vi "LVDemo2.vi"() -> ()   [LabVIEW 2010]
uses:
  toupcam.dll
  toupcam_labview.dll
panel:
  in  "Tab 2":T1(tab)
  in  "Color Default 2":bool
  in  "Brightness 2":i32(slide) scale=-64.0..64.0
  in  "Contrast 2":i32(slide) scale=-100.0..100.0
  in  "Gamma 2":i32(slide) scale=20.0..180.0
  in  "Hue 2":i32(slide) scale=-180.0..180.0
  in  "Saturation 2":i32(slide) scale=0.0..255.0
  in  "AutoExpo 2":bool
  in  "ExpoDefault 2":bool
  in  "Expotime 2":u32(slide)
  in  "ExpoGain 2":u16(slide)
  in  "AutoWB 2":bool
  in  "WBDefault 2":bool
  in  "Tint 2":i32(slide) scale=200.0..2500.0
  in  "Temp 2":i32(slide) scale=2000.0..15000.0
  in  "Bin/Skip Mode 2":bool
  in  "Chrome/Mono 2":bool
  in  "HFlip 2":bool
  in  "VFlip 2":bool
  in  "Frame Speed 2":u8(slide) scale=0.0..87.0
  in  "Cap Still Image 2":bool
  in  "Still Image Resolution 2":u16(ring)
  in  "Cap Live Image 2":bool
  in  "Live Resolution 2":u16(ring)
  out "Video 2":T2(plugin-control)
  in  "Tab":T1(tab)
  in  "Color Default":bool
  in  "Brightness":i32(slide) scale=-64.0..64.0
  in  "Contrast":i32(slide) scale=-100.0..100.0
  in  "Gamma":i32(slide) scale=20.0..180.0
  in  "Hue":i32(slide) scale=-180.0..180.0
  in  "Saturation":i32(slide) scale=0.0..255.0
  in  "AutoExpo":bool
  in  "ExpoDefault":bool
  in  "Expotime":u32(slide) scale=294.0..2000000.0
  in  "ExpoGain":u16(slide) scale=100.0..300.0
  in  "AutoWB":bool
  in  "WBDefault":bool
  in  "Tint":i32(slide) scale=200.0..2500.0
  in  "Temp":i32(slide) scale=2000.0..15000.0
  in  "Bin/Skip Mode":bool
  in  "Chrome/Mono":bool
  in  "HFlip":bool
  in  "VFlip":bool
  in  "Frame Speed":u8(slide) scale=0.0..6.0
  out "Video":T2(plugin-control)
  in  "Cap Still Image":bool
  in  "Still Image Resolution":u16(ring) items=["2592*1944", "1280*960", "640*480"]
  in  "Cap Live Image":bool
  in  "Stop":bool
  in  "Live Resolution":u16(ring) items=["2592*1944", "1280*960", "640*480"]
  in  "?":enum32{"选项卡 1"}(tab)
  in  "Expotime_def 2":u32
  in  "ExpoGain_def 2":u16
  in  "ExpoGain_Max 2":u16
  in  "ExpoGain_Min 2":u16
  in  "Height 2":i32
  in  "Width 2":i32
  in  "Expotime_Max 2":u32
  in  "Expotime_Min 2":u32
  in  "speed 2":u8
  in  "height22":i32
  in  "width22":i32
  in  "Mode 2":bool
  in  "Expotime_def":u32
  in  "ExpoGain_def":u16
  in  "ExpoGain_Max":u16
  in  "ExpoGain_Min":u16
  in  "Height":i32
  in  "Width":i32
  in  "Expotime_Max":u32
  in  "Expotime_Min":u32
  in  "speed":u8
  in  "height12":i32
  in  "width12":i32
  in  "Mode":bool
  in  "Still_Height 3":i32
  in  "Still_Width 3":i32
  in  "ExpoGain 5":u16
  in  "Expotime 5":u32
  in  "Tint 5":i32
  in  "Temp 5":i32
  in  "ExpoGain 6":u16
  in  "Expotime 6":u32
  in  "Temp 6":i32
  in  "Tint 6":i32
  in  "Still_Width 4":i32
  in  "Still_Height 4":i32
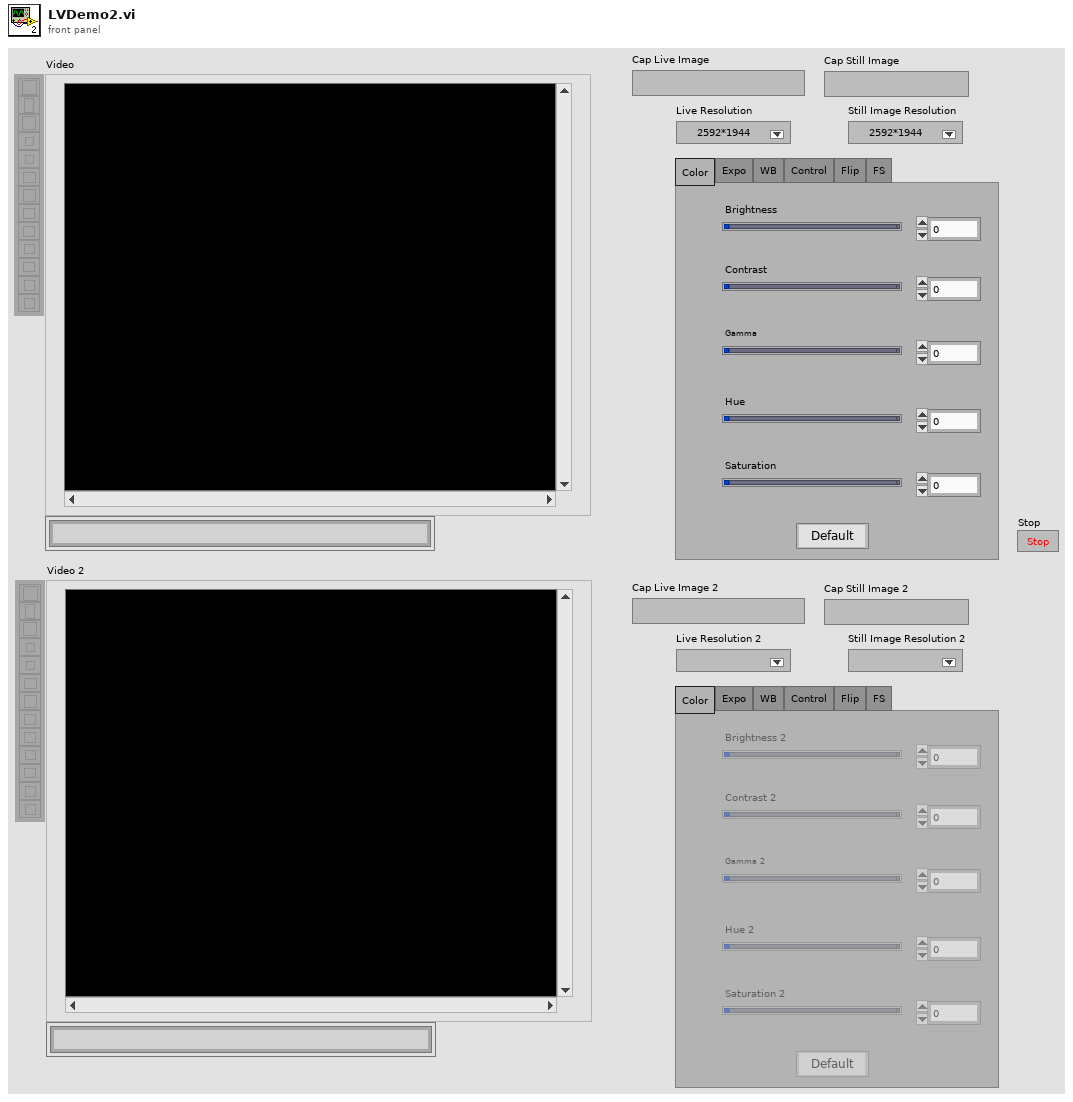
[diagram p1: front panel]
types:
  T1 = enum32{"Color", "Expo", "WB", "Control", "Flip", "FS"}
  T2 = typedef "IMAQ Image.ctl" = refnum<image>
  T3 = enum8{"Enabled", "Disabled", "Disabled and Grayed Out"}
  T4 = typedef "Image Type" = u32
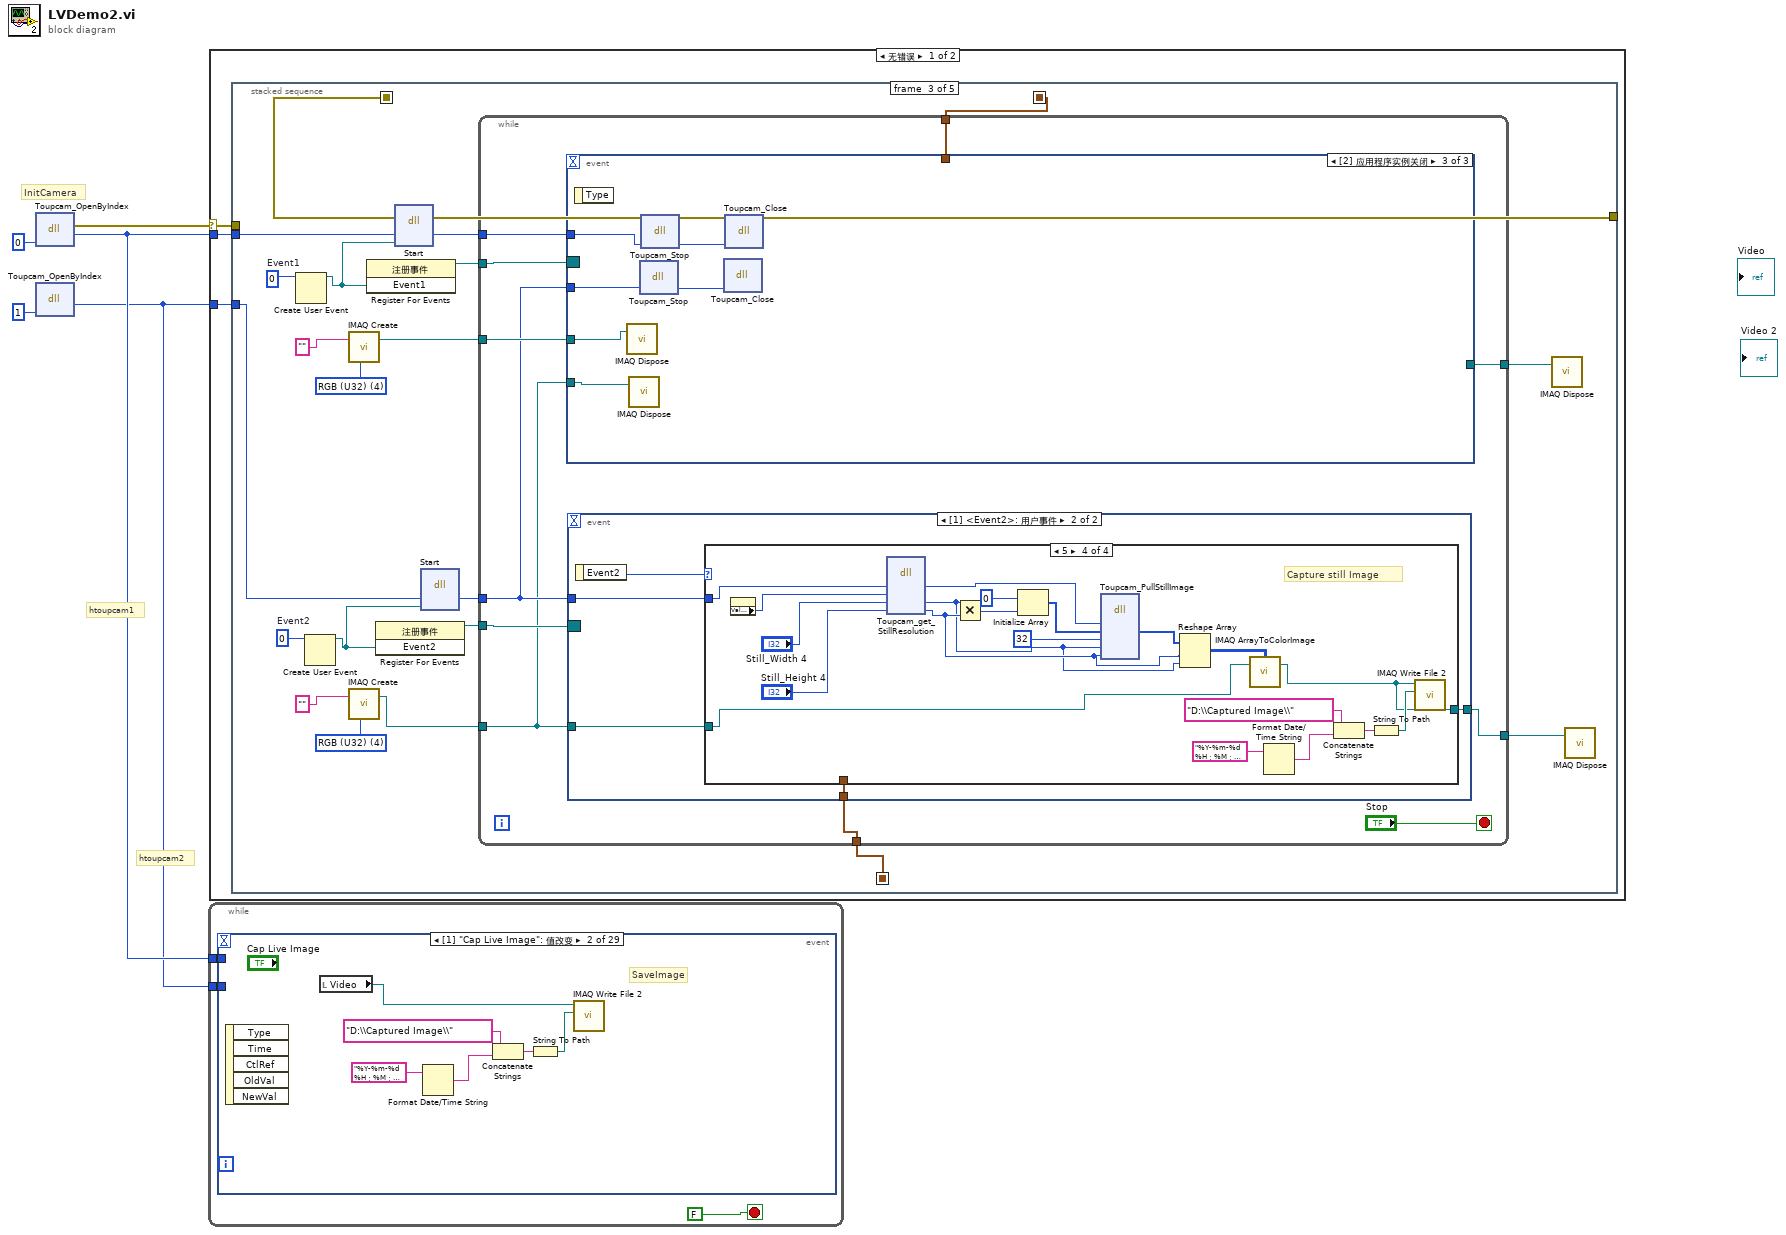
[diagram p0: block diagram]
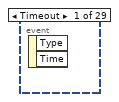
[diagram p2: hidden frame]
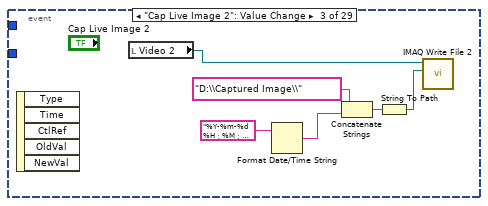
[diagram p3: hidden frame]
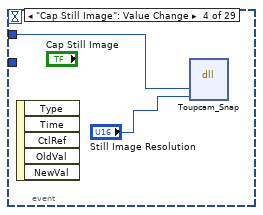
[diagram p4: hidden frame]
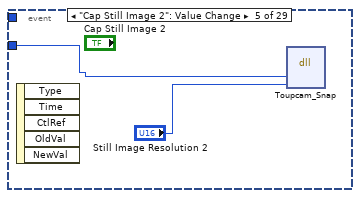
[diagram p5: hidden frame]
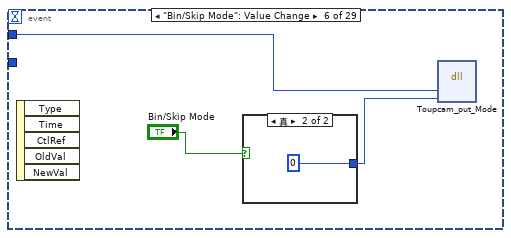
[diagram p6: hidden frame]
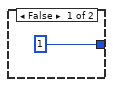
[diagram p7: hidden frame]
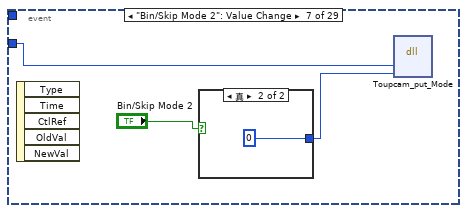
[diagram p8: hidden frame]
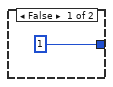
[diagram p9: hidden frame]
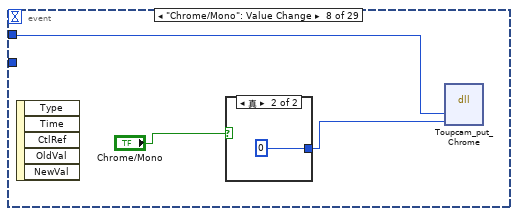
[diagram p10: hidden frame]
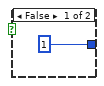
[diagram p11: hidden frame]
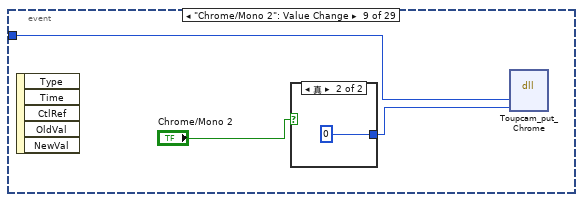
[diagram p12: hidden frame]
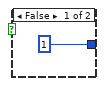
[diagram p13: hidden frame]
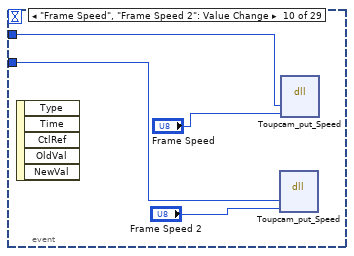
[diagram p14: hidden frame]
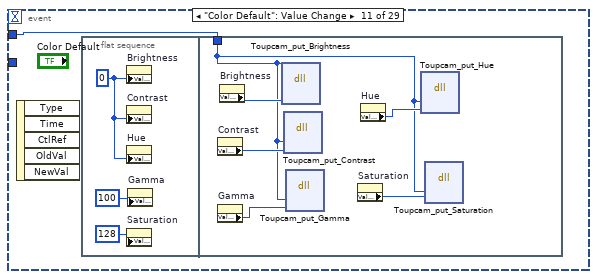
[diagram p15: hidden frame]
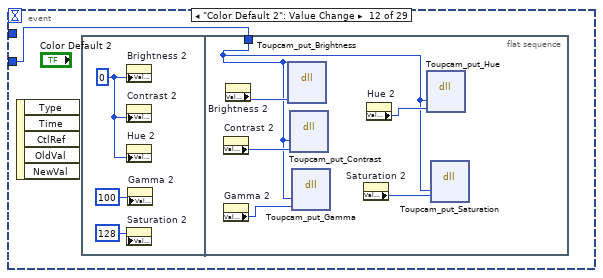
[diagram p16: hidden frame]
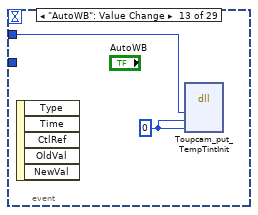
[diagram p17: hidden frame]
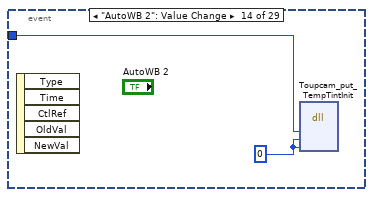
[diagram p18: hidden frame]
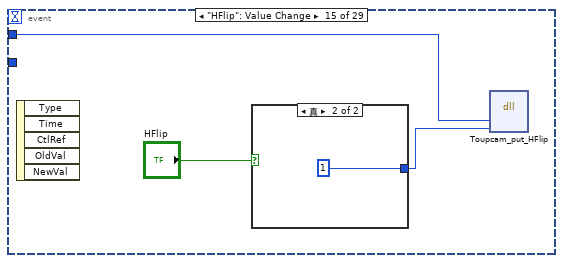
[diagram p19: hidden frame]
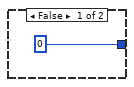
[diagram p20: hidden frame]
diagram:
  # "htoupcam1"
  # "htoupcam2"
  # "InitCamera"
  n1 = dll-call lib="C:/LVDemo x86/toupcam.dll" fn="Toupcam_OpenByIndex"("Index"=0) -> (error out=w4:errorcluster, "返回类型"=w3:i32)  [unwired: 4 in, 1 out]
  n2 = dll-call lib="C:/LVDemo x86/toupcam.dll" fn="Toupcam_OpenByIndex"("Index"=1) -> ("return type"=w1:i32)  [unwired: 4 in, 2 out]
  n3 = while {
    tunnel: w3 -> [w7]
    tunnel: w1 -> [w6]
    stop <- FALSE ("停止 2") stop-if-true
    n4 = event shown="[1] \"Cap Live Image\": 值改变" {
      selector: _ -> [_ _ _ _ _ _ _ _ _ _ _ _ _ _ _ _ _ _ _ _ _ _ _ _ _ _ _ _ _]
      dyn-events: _ -> [_ _ _ _ _ _ _ _ _ _ _ _ _ _ _ _ _ _ _ _ _ _ _ _ _ _ _ _ _]
      timeout: _ -> [_ _ _ _ _ _ _ _ _ _ _ _ _ _ _ _ _ _ _ _ _ _ _ _ _ _ _ _ _]
      tunnel: w7 -> [_ _ _ w22 _ w27 _ w37 _ w47 w49 _ w70 _ w75 _ w85 _ w96 _ w110 _ w139 w145 w152 _ w167 w171 w178]
      tunnel: w6 -> [_ _ _ _ w24 _ w31 _ w40 w45 _ w59 _ w71 _ w78 _ w88 _ w101 _ w124 _ _ _ w161 w165 w169 w175]
      event Timeout {
        n5 = event-data() -> ()  [unwired: 1 in, 2 out]
      }
      event "Cap Live Image": Value Change {
        # "SaveImage"
        n6 = event-data() -> ()  [unwired: 1 in, 5 out]
        n7 = local read "Video"() -> (w9:T2)
        n8 = Format Date/Time String(time format string (%c)="%Y-%m-%d %H：%M：%S.bmp ") -> (date/time string=w13:string)  [unwired: 2 in]
        n9 = Concatenate Strings("D:\\Captured Image\\", w13) -> (w10:string)
        n10 = String To Path(string=w10) -> (path=w12:path)
        n11 = call-poly "IMAQ Write File 2"("File Path"=w12, "Image"=w9) -> ()  [unwired: 8 in, 2 out]
      }
      event "Cap Live Image 2": Value Change {
        n12 = event-data() -> ()  [unwired: 1 in, 5 out]
        n13 = local read "Video 2"() -> (w15:T2)
        n14 = Format Date/Time String(time format string (%c)="%Y-%m-%d %H：%M：%S.bmp ") -> (date/time string=w19:string)  [unwired: 2 in]
        n15 = Concatenate Strings("D:\\Captured Image\\", w19) -> (w16:string)
        n16 = String To Path(string=w16) -> (path=w18:path)
        n17 = call-poly "IMAQ Write File 2"("File Path"=w18, "Image"=w15) -> ()  [unwired: 8 in, 2 out]
      }
      event "Cap Still Image": Value Change {
        n18 = event-data() -> ()  [unwired: 1 in, 5 out]
        n19 = dll-call lib="C:/LVDemo x86/toupcam.dll" fn="Toupcam_Snap"("htoupcam"=w22, "ResIndex"="Still Image Resolution") -> ()  [unwired: 6 in, 2 out]
      }
      event "Cap Still Image 2": Value Change {
        n20 = event-data() -> ()  [unwired: 1 in, 5 out]
        n21 = dll-call lib="C:/LVDemo x86/toupcam.dll" fn="Toupcam_Snap"("htoupcam"=w24, "ResIndex"="Still Image Resolution 2") -> ()  [unwired: 6 in, 2 out]
      }
      event "Bin/Skip Mode": Value Change {
        n22 = event-data() -> ()  [unwired: 1 in, 5 out]
        n23 = case shown="真" "Bin/Skip Mode" {
          tunnel: [1 0] -> w25
          frame False {
          }
          frame True {
          }
        }
        n24 = dll-call lib="C:/LVDemo x86/toupcam.dll" fn="Toupcam_put_Mode"("htoupcam"=w27, "mode"=w25) -> ()  [unwired: 6 in, 2 out]
      }
      event "Bin/Skip Mode 2": Value Change {
        n25 = event-data() -> ()  [unwired: 1 in, 5 out]
        n26 = case shown="真" "Bin/Skip Mode 2" {
          tunnel: [1 0] -> w32
          frame False {
          }
          frame True {
          }
        }
        n27 = dll-call lib="C:/LVDemo x86/toupcam.dll" fn="Toupcam_put_Mode"("htoupcam"=w31, "mode"=w32) -> ()  [unwired: 6 in, 2 out]
      }
      event "Chrome/Mono": Value Change {
        n28 = event-data() -> ()  [unwired: 1 in, 5 out]
        n29 = case shown="真" "Chrome/Mono" {
          tunnel: [1 0] -> w35
          frame False {
          }
          frame True {
          }
        }
        n30 = dll-call lib="C:/LVDemo x86/toupcam.dll" fn="Toupcam_put_Chrome"("htoupcam"=w37, "chrome"=w35) -> ()  [unwired: 6 in, 2 out]
      }
      event "Chrome/Mono 2": Value Change {
        n31 = event-data() -> ()  [unwired: 1 in, 5 out]
        n32 = case shown="真" "Chrome/Mono 2" {
          tunnel: [1 0] -> w42
          frame False {
          }
          frame True {
          }
        }
        n33 = dll-call lib="C:/LVDemo x86/toupcam.dll" fn="Toupcam_put_Chrome"("htoupcam"=w40, "chrome"=w42) -> ()  [unwired: 6 in, 2 out]
      }
      event "Frame Speed", "Frame Speed 2": Value Change {
        n34 = event-data() -> ()  [unwired: 1 in, 5 out]
        n35 = dll-call lib="C:/LVDemo x86/toupcam.dll" fn="Toupcam_put_Speed"("htoupcam"=w45, "Speed"="Frame Speed 2") -> ()  [unwired: 6 in, 2 out]
        n36 = dll-call lib="C:/LVDemo x86/toupcam.dll" fn="Toupcam_put_Speed"("htoupcam"=w47, "Speed"="Frame Speed") -> ()  [unwired: 6 in, 2 out]
      }
      event "Color Default": Value Change {
        n37 = event-data() -> ()  [unwired: 1 in, 5 out]
        n38 = flat-sequence {
          tunnel: w49 -> [w53]
          frame #0 {
            w52 = 0
            n39 = property on="Brightness" class="Slide (严格)"("Value"=w52) -> ()  [unwired: 2 in, 2 out]
            n40 = property on="Contrast" class="Slide (严格)"("Value"=w52) -> ()  [unwired: 2 in, 2 out]
            n41 = property on="Hue" class="Slide (严格)"("Value"=w52) -> ()  [unwired: 2 in, 2 out]
            n42 = property on="Saturation" class="Slide (严格)"("Value"=128) -> ()  [unwired: 2 in, 2 out]
            n43 = property on="Gamma" class="Slide (严格)"("Value"=100) -> ()  [unwired: 2 in, 2 out]
          }
          frame #1 {
            n44 = property on="Contrast" class="Slide (严格)"() -> ("Value"=w57:i32)  [unwired: 2 in, 2 out]
            n45 = property on="Gamma" class="Slide (严格)"() -> ("Value"=w56:i32)  [unwired: 2 in, 2 out]
            n46 = property on="Brightness" class="Slide (严格)"() -> ("Value"=w58:i32)  [unwired: 2 in, 2 out]
            n47 = dll-call lib="C:/LVDemo x86/toupcam.dll" fn="Toupcam_put_Brightness"("htoupcam"=w53, "Brightness"=w58) -> ()  [unwired: 6 in, 2 out]
            n48 = dll-call lib="C:/LVDemo x86/toupcam.dll" fn="Toupcam_put_Contrast"("htoupcam"=w53, "Contrast"=w57) -> ()  [unwired: 6 in, 2 out]
            n49 = dll-call lib="C:/LVDemo x86/toupcam.dll" fn="Toupcam_put_Gamma"("htoupcam"=w53, "Gamma"=w56) -> ()  [unwired: 6 in, 2 out]
            n50 = property on="Saturation" class="Slide (严格)"() -> ("Value"=w54:i32)  [unwired: 2 in, 2 out]
            n51 = property on="Hue" class="Slide (严格)"() -> ("Value"=w55:i32)  [unwired: 2 in, 2 out]
            n52 = dll-call lib="C:/LVDemo x86/toupcam.dll" fn="Toupcam_put_Hue"("htoupcam"=w53, "Hue"=w55) -> ()  [unwired: 6 in, 2 out]
            n53 = dll-call lib="C:/LVDemo x86/toupcam.dll" fn="Toupcam_put_Saturation"("htoupcam"=w53, "Saturation"=w54) -> ()  [unwired: 6 in, 2 out]
          }
        }
      }
      event "Color Default 2": Value Change {
        n54 = event-data() -> ()  [unwired: 1 in, 5 out]
        n55 = flat-sequence {
          tunnel: w59 -> [w63]
          frame #0 {
            w62 = 0
            n56 = property on="Brightness 2" class="Slide (严格)"("Value"=w62) -> ()  [unwired: 2 in, 2 out]
            n57 = property on="Contrast 2" class="Slide (严格)"("Value"=w62) -> ()  [unwired: 2 in, 2 out]
            n58 = property on="Hue 2" class="Slide (严格)"("Value"=w62) -> ()  [unwired: 2 in, 2 out]
            n59 = property on="Saturation 2" class="Slide (严格)"("Value"=128) -> ()  [unwired: 2 in, 2 out]
            n60 = property on="Gamma 2" class="Slide (严格)"("Value"=100) -> ()  [unwired: 2 in, 2 out]
          }
          frame #1 {
            n61 = property on="Contrast 2" class="Slide (严格)"() -> ("Value"=w67:i32)  [unwired: 2 in, 2 out]
            n62 = property on="Gamma 2" class="Slide (严格)"() -> ("Value"=w66:i32)  [unwired: 2 in, 2 out]
            n63 = property on="Brightness 2" class="Slide (严格)"() -> ("Value"=w68:i32)  [unwired: 2 in, 2 out]
            n64 = dll-call lib="C:/LVDemo x86/toupcam.dll" fn="Toupcam_put_Brightness"("htoupcam"=w63, "Brightness"=w68) -> ()  [unwired: 6 in, 2 out]
            n65 = dll-call lib="C:/LVDemo x86/toupcam.dll" fn="Toupcam_put_Contrast"("htoupcam"=w63, "Contrast"=w67) -> ()  [unwired: 6 in, 2 out]
            n66 = dll-call lib="C:/LVDemo x86/toupcam.dll" fn="Toupcam_put_Gamma"("htoupcam"=w63, "Gamma"=w66) -> ()  [unwired: 6 in, 2 out]
            n67 = property on="Saturation 2" class="Slide (严格)"() -> ("Value"=w64:i32)  [unwired: 2 in, 2 out]
            n68 = property on="Hue 2" class="Slide (严格)"() -> ("Value"=w65:i32)  [unwired: 2 in, 2 out]
            n69 = dll-call lib="C:/LVDemo x86/toupcam.dll" fn="Toupcam_put_Hue"("htoupcam"=w63, "Hue"=w65) -> ()  [unwired: 6 in, 2 out]
            n70 = dll-call lib="C:/LVDemo x86/toupcam.dll" fn="Toupcam_put_Saturation"("htoupcam"=w63, "Saturation"=w64) -> ()  [unwired: 6 in, 2 out]
          }
        }
      }
      event "AutoWB": Value Change {
        w69 = 0
        n71 = event-data() -> ()  [unwired: 1 in, 5 out]
        n72 = dll-call lib="C:/LVDemo x86/toupcam.dll" fn="Toupcam_put_TempTintInit"("htoupcam"=w70, "fnTTProc"=w69, "pTTCtx"=w69) -> ()  [unwired: 7 in, 2 out]
      }
      event "AutoWB 2": Value Change {
        w72 = 0
        n73 = event-data() -> ()  [unwired: 1 in, 5 out]
        n74 = dll-call lib="C:/LVDemo x86/toupcam.dll" fn="Toupcam_put_TempTintInit"("htoupcam"=w71, "fnTTProc"=w72, "pTTCtx"=w72) -> ()  [unwired: 7 in, 2 out]
      }
      event "HFlip": Value Change {
        n75 = event-data() -> ()  [unwired: 1 in, 5 out]
        n76 = case shown="真" "HFlip" {
          tunnel: [0 1] -> w73
          frame False {
          }
          frame True {
          }
        }
        n77 = dll-call lib="C:/LVDemo x86/toupcam.dll" fn="Toupcam_put_HFlip"("htoupcam"=w75, "bHFlip"=w73) -> ()  [unwired: 6 in, 2 out]
      }
      event "HFlip 2": Value Change {
        n78 = event-data() -> ()  [unwired: 1 in, 5 out]
        n79 = case shown="真" "HFlip 2" {
          tunnel: [0 1] -> w80
          frame False {
          }
          frame True {
          }
        }
        n80 = dll-call lib="C:/LVDemo x86/toupcam.dll" fn="Toupcam_put_HFlip"("htoupcam"=w78, "bHFlip"=w80) -> ()  [unwired: 6 in, 2 out]
      }
      event "VFlip": Value Change {
        n81 = event-data() -> ()  [unwired: 1 in, 5 out]
        n82 = case shown="真" "VFlip" {
          tunnel: [0 1] -> w83
          frame False {
          }
          frame True {
          }
        }
        n83 = dll-call lib="C:/LVDemo x86/toupcam.dll" fn="Toupcam_put_VFlip"("htoupcam"=w85, "bVFlip"=w83) -> ()  [unwired: 6 in, 2 out]
      }
      event "VFlip 2": Value Change {
        n84 = event-data() -> ()  [unwired: 1 in, 5 out]
        n85 = case shown="真" "VFlip 2" {
          tunnel: [0 1] -> w90
          frame False {
          }
          frame True {
          }
        }
        n86 = dll-call lib="C:/LVDemo x86/toupcam.dll" fn="Toupcam_put_VFlip"("htoupcam"=w88, "bVFlip"=w90) -> ()  [unwired: 6 in, 2 out]
      }
      event "AutoExpo": Value Change {
        n87 = event-data() -> ()  [unwired: 1 in, 5 out]
        n88 = case shown="假" "AutoExpo" {
          tunnel: [0 1] -> w95
          tunnel: [T3."Enabled" ("禁用") T3."Disabled and Grayed Out" ("禁用")] -> w93
          frame False {
          }
          frame True {
          }
        }
        n89 = dll-call lib="C:/LVDemo x86/toupcam.dll" fn="Toupcam_put_AutoExpoEnable"("HToupcam"=w96, "bAutoExposure"=w95) -> ()  [unwired: 6 in, 2 out]
        n90 = property on="Expotime" class="Slide (严格)"("DisabledEnum"=w93) -> ()  [unwired: 2 in, 2 out]
        n91 = property on="ExpoGain" class="Slide (严格)"("DisabledEnum"=w93) -> ()  [unwired: 2 in, 2 out]
      }
      event "AutoExpo 2": Value Change {
        n92 = event-data() -> ()  [unwired: 1 in, 5 out]
        n93 = case shown="假" "AutoExpo 2" {
          tunnel: [0 1] -> w104
          tunnel: [T3."Enabled" ("禁用") T3."Disabled and Grayed Out" ("禁用")] -> w103
          frame False {
          }
          frame True {
          }
        }
        n94 = dll-call lib="C:/LVDemo x86/toupcam.dll" fn="Toupcam_put_AutoExpoEnable"("HToupcam"=w101, "bAutoExposure"=w104) -> ()  [unwired: 6 in, 2 out]
        n95 = property on="Expotime 2" class="Slide (严格)"("DisabledEnum"=w103) -> ()  [unwired: 2 in, 2 out]
        n96 = property on="ExpoGain 2" class="Slide (严格)"("DisabledEnum"=w103) -> ()  [unwired: 2 in, 2 out]
      }
      event "ExpoDefault": Value Change {
        n97 = event-data() -> ()  [unwired: 1 in, 5 out]
        n98 = flat-sequence {
          tunnel: w110 -> [w112]
          tunnel: [w111] -> w109
          tunnel: w109 -> [w121]
          frame #0 {
            n99 = local read "Expotime_def"() -> (w118:u32)
            n100 = local read "ExpoGain_def"() -> (w114:u16)
            n101 = local read "ExpoGain_Min"() -> (w120:u16)
            n102 = local read "ExpoGain_Min"() -> (w116:u16)
            n103 = local read "Expotime_Max"() -> (w119:u32)
            n104 = local read "ExpoGain_Max"() -> (w115:u16)
            n105 = dll-call lib="C:/LVDemo x86/toupcam.dll" fn="Toupcam_get_ExpoAGainRange"("htoupcam"=w112, "min"=w116, "max"=w115, "def"=w114) -> ("def"=w117:u16)  [unwired: 7 in, 2 out]
            n106 = dll-call lib="C:/LVDemo x86/toupcam.dll" fn="Toupcam_get_ExpTimeRange"("htoupcam"=w112, "Min"=w120, "Max"=w119, "def"=w118) -> ("htoupcam"=w111:i32, "def"=w113:u32)  [unwired: 6 in, 2 out]
            n107 = property on="Expotime" class="Slide (严格)"("Value"=w113) -> ()  [unwired: 2 in, 2 out]
            n108 = property on="ExpoGain" class="Slide (严格)"("Value"=w117) -> ()  [unwired: 2 in, 2 out]
          }
          frame #1 {
            n109 = property on="Expotime" class="Slide (严格)"() -> ("Value"=w123:u32)  [unwired: 2 in, 2 out]
            n110 = property on="ExpoGain" class="Slide (严格)"() -> ("Value"=w122:u16)  [unwired: 2 in, 2 out]
            n111 = dll-call lib="C:/LVDemo x86/toupcam.dll" fn="Toupcam_put_ExpoTime"("htoupcam"=w121, "Expotime"=w123) -> ()  [unwired: 6 in, 2 out]
            n112 = dll-call lib="C:/LVDemo x86/toupcam.dll" fn="Toupcam_put_ExpoAGain"("htoupcam"=w121, "ExpoGain"=w122) -> ()  [unwired: 6 in, 2 out]
          }
        }
      }
      event "ExpoDefault 2": Value Change {
        n113 = event-data() -> ()  [unwired: 1 in, 5 out]
        n114 = flat-sequence {
          tunnel: w124 -> [w127]
          tunnel: [w126] -> w125
          tunnel: w125 -> [w136]
          frame #0 {
            n115 = local read "Expotime_def 2"() -> (w133:u32)
            n116 = local read "ExpoGain_def 2"() -> (w129:u16)
            n117 = local read "Expotime_Min 2"() -> (w135:u32)
            n118 = local read "ExpoGain_Min 2"() -> (w131:u16)
            n119 = local read "Expotime_Max 2"() -> (w134:u32)
            n120 = local read "ExpoGain_Max 2"() -> (w130:u16)
            n121 = dll-call lib="C:/LVDemo x86/toupcam.dll" fn="Toupcam_get_ExpoAGainRange"("htoupcam"=w127, "min"=w131, "max"=w130, "def"=w129) -> ("def"=w132:u16)  [unwired: 7 in, 2 out]
            n122 = dll-call lib="C:/LVDemo x86/toupcam.dll" fn="Toupcam_get_ExpTimeRange"("htoupcam"=w127, "Min"=w135, "Max"=w134, "def"=w133) -> ("htoupcam"=w126:i32, "def"=w128:u32)  [unwired: 6 in, 2 out]
            n123 = property on="Expotime 2" class="Slide (严格)"("Value"=w128) -> ()  [unwired: 2 in, 2 out]
            n124 = property on="ExpoGain 2" class="Slide (严格)"("Value"=w132) -> ()  [unwired: 2 in, 2 out]
          }
          frame #1 {
            n125 = property on="Expotime 2" class="Slide (严格)"() -> ("Value"=w138:u32)  [unwired: 2 in, 2 out]
            n126 = property on="ExpoGain 2" class="Slide (严格)"() -> ("Value"=w137:u16)  [unwired: 2 in, 2 out]
            n127 = dll-call lib="C:/LVDemo x86/toupcam.dll" fn="Toupcam_put_ExpoTime"("htoupcam"=w136, "Expotime"=w138) -> ()  [unwired: 6 in, 2 out]
            n128 = dll-call lib="C:/LVDemo x86/toupcam.dll" fn="Toupcam_put_ExpoAGain"("htoupcam"=w136, "ExpoGain"=w137) -> ()  [unwired: 6 in, 2 out]
          }
        }
      }
      event "WBDefault": Value Change {
        n129 = event-data() -> ()  [unwired: 1 in, 5 out]
        n130 = flat-sequence {
          tunnel: w139 -> [w144]
          frame #0 {
            n131 = property on="Temp" class="Slide (严格)"("Value"=6503) -> ()  [unwired: 2 in, 2 out]
            n132 = property on="Tint" class="Slide (严格)"("Value"=1000) -> ()  [unwired: 2 in, 2 out]
          }
          frame #1 {
            n133 = property on="Temp" class="Slide (严格)"() -> ("Value"=w143:i32)  [unwired: 2 in, 2 out]
            n134 = property on="Tint" class="Slide (严格)"() -> ("Value"=w142:i32)  [unwired: 2 in, 2 out]
            n135 = dll-call lib="C:/LVDemo x86/toupcam.dll" fn="Toupcam_put_TempTint"("htoupcam"=w144, "Temp"=w143, "Tint"=w142) -> ()  [unwired: 7 in, 2 out]
          }
        }
      }
      event "WBDefault 2": Value Change {
        n136 = event-data() -> ()  [unwired: 1 in, 5 out]
        n137 = flat-sequence {
          tunnel: w145 -> [w150]
          frame #0 {
            n138 = property on="Temp 2" class="Slide (严格)"("Value"=6503) -> ()  [unwired: 2 in, 2 out]
            n139 = property on="Tint 2" class="Slide (严格)"("Value"=1000) -> ()  [unwired: 2 in, 2 out]
          }
          frame #1 {
            n140 = property on="Temp 2" class="Slide (严格)"() -> ("Value"=w149:i32)  [unwired: 2 in, 2 out]
            n141 = property on="Tint 2" class="Slide (严格)"() -> ("Value"=w148:i32)  [unwired: 2 in, 2 out]
            n142 = dll-call lib="C:/LVDemo x86/toupcam.dll" fn="Toupcam_put_TempTint"("htoupcam"=w150, "Temp"=w149, "Tint"=w148) -> ()  [unwired: 7 in, 2 out]
          }
        }
      }
      event "Brightness", "Contrast", "Gamma", "Hue", "Saturation": Value Change {
        n143 = event-data() -> ()  [unwired: 1 in, 5 out]
        n144 = dll-call lib="C:/LVDemo x86/toupcam.dll" fn="Toupcam_put_Brightness"("htoupcam"=w152, "Brightness"="Brightness") -> ("htoupcam"=w151:i32)  [unwired: 5 in, 2 out]
        n145 = dll-call lib="C:/LVDemo x86/toupcam.dll" fn="Toupcam_put_Contrast"("htoupcam"=w152, "Contrast"="Contrast") -> ()  [unwired: 6 in, 2 out]
        n146 = dll-call lib="C:/LVDemo x86/toupcam.dll" fn="Toupcam_put_Gamma"("htoupcam"=w152, "Gamma"="Gamma") -> ()  [unwired: 6 in, 2 out]
        n147 = dll-call lib="C:/LVDemo x86/toupcam.dll" fn="Toupcam_put_Hue"("htoupcam"=w151, "Hue"="Hue") -> ()  [unwired: 6 in, 2 out]
        n148 = dll-call lib="C:/LVDemo x86/toupcam.dll" fn="Toupcam_put_Saturation"("htoupcam"=w151, "Saturation"="Saturation") -> ()  [unwired: 6 in, 2 out]
      }
      event "Brightness 2", "Contrast 2", "Gamma 2", "Hue 2", "Saturation 2": Value Change {
        n149 = event-data() -> ()  [unwired: 1 in, 5 out]
        n150 = dll-call lib="C:/LVDemo x86/toupcam.dll" fn="Toupcam_put_Brightness"("htoupcam"=w161, "Brightness"="Brightness 2") -> ("htoupcam"=w158:i32)  [unwired: 5 in, 2 out]
        n151 = dll-call lib="C:/LVDemo x86/toupcam.dll" fn="Toupcam_put_Contrast"("htoupcam"=w161, "Contrast"="Contrast 2") -> ()  [unwired: 6 in, 2 out]
        n152 = dll-call lib="C:/LVDemo x86/toupcam.dll" fn="Toupcam_put_Gamma"("htoupcam"=w161, "Gamma"="Gamma 2") -> ()  [unwired: 6 in, 2 out]
        n153 = dll-call lib="C:/LVDemo x86/toupcam.dll" fn="Toupcam_put_Hue"("htoupcam"=w158, "Hue"="Hue 2") -> ()  [unwired: 6 in, 2 out]
        n154 = dll-call lib="C:/LVDemo x86/toupcam.dll" fn="Toupcam_put_Saturation"("htoupcam"=w158, "Saturation"="Saturation 2") -> ()  [unwired: 6 in, 2 out]
      }
      event "Expotime", "Expotime 2": Value Change {
        n155 = event-data() -> ()  [unwired: 1 in, 5 out]
        n156 = dll-call lib="C:/LVDemo x86/toupcam.dll" fn="Toupcam_put_ExpoTime"("htoupcam"=w167, "Expotime"="Expotime") -> ()  [unwired: 6 in, 2 out]
        n157 = dll-call lib="C:/LVDemo x86/toupcam.dll" fn="Toupcam_put_ExpoTime"("htoupcam"=w165, "Expotime"="Expotime 2") -> ()  [unwired: 6 in, 2 out]
      }
      event "ExpoGain", "ExpoGain 2": Value Change {
        n158 = event-data() -> ()  [unwired: 1 in, 5 out]
        n159 = dll-call lib="C:/LVDemo x86/toupcam.dll" fn="Toupcam_put_ExpoAGain"("htoupcam"=w171, "ExpoGain"="ExpoGain") -> ()  [unwired: 6 in, 2 out]
        n160 = dll-call lib="C:/LVDemo x86/toupcam.dll" fn="Toupcam_put_ExpoAGain"("htoupcam"=w169, "ExpoGain"="ExpoGain 2") -> ()  [unwired: 6 in, 2 out]
      }
      event "Temp", "Tint", "Temp 2", "Tint 2": Value Change {
        n161 = event-data() -> ()  [unwired: 1 in, 5 out]
        n162 = dll-call lib="C:/LVDemo x86/toupcam.dll" fn="Toupcam_put_TempTint"("htoupcam"=w178, "Temp"="Temp", "Tint"="Tint") -> ()  [unwired: 7 in, 2 out]
        n163 = dll-call lib="C:/LVDemo x86/toupcam.dll" fn="Toupcam_put_TempTint"("htoupcam"=w175, "Temp"="Temp 2", "Tint"="Tint 2") -> ()  [unwired: 7 in, 2 out]
      }
    }
  }
  n164 = case shown="无错误" w4 {
    selector: w4 -> [w180 _]
    tunnel: w3 -> [w181 _]
    tunnel: w1 -> [w179 _]
    frame No Error {
      n165 = stacked-sequence {
        seq-local: [w231 _ _ _ _] -> [_ _ w305 _ _]
        seq-local: [w230 _ _ _ _] -> [_ _ w304 _ _]
        seq-local: [w213 _ _ _ _] -> [_ _ w299 _ _]
        tunnel: w181 -> [w219 _ w309 w422 w426]
        tunnel: w180 -> [w230 _ _ _ w425]
        tunnel: [_ _ w303 _ _] -> _
        tunnel: w179 -> [w200 _ w301 w421 w423]
        frame #0 {
          # "SetSliderRange"
          # "SetCameraResolution"
          # "CameraResolution"
          n166 = dll-call lib="C:/LVDemo x86/toupcam.dll" fn="Toupcam_get_ExpTimeRange"("htoupcam"=w219, "Min"="Expotime_Min", "Max"="Expotime_Max", "def"="Expotime_def") -> ("Min"=w234:u32, "Max"=w233:u32, "def"=w232:u32)  [unwired: 5 in, 2 out]
          n167 = dll-call lib="C:/LVDemo x86/toupcam.dll" fn="Toupcam_get_ExpoAGainRange"("htoupcam"=w219, "min"="ExpoGain_Min", "max"="ExpoGain_Max", "def"="ExpoGain_def") -> ("min"=w241:u16, "max"=w240:u16, "def"=w239:u16)  [unwired: 5 in, 2 out]
          n168 = dll-call lib="C:/LVDemo x86/toupcam.dll" fn="Toupcam_put_AutoExpoEnable"("htoupcam"=w200, "bAutoExposure"=FALSE) -> ()  [unwired: 6 in, 2 out]
          n169 = dll-call lib="C:/LVDemo x86/toupcam.dll" fn="Toupcam_put_ExpoTime"("htoupcam"=w200, "Time"=5000) -> ("htoupcam"=w197:i32)  [unwired: 5 in, 2 out]
          n170 = dll-call lib="C:/LVDemo x86/toupcam.dll" fn="Toupcam_get_ExpTimeRange"("htoupcam"=w200, "Min"="Expotime_Min 2", "Max"="Expotime_Max 2", "def"="Expotime_def 2") -> ("Min"=w207:u32, "Max"=w206:u32, "def"=w205:u32)  [unwired: 5 in, 2 out]
          n171 = dll-call lib="C:/LVDemo x86/toupcam.dll" fn="Toupcam_get_ExpoAGainRange"("htoupcam"=w200, "min"="ExpoGain_Min 2", "max"="ExpoGain_Max 2", "def"="ExpoGain_def 2") -> ("min"=w204:u16, "max"=w203:u16, "def"=w202:u16)  [unwired: 5 in, 2 out]
          n172 = dll-call lib="C:/LVDemo x86/toupcam.dll" fn="Toupcam_put_AutoExpoEnable"("htoupcam"=w219, "bAutoExposure"=FALSE) -> ()  [unwired: 6 in, 2 out]
          n173 = dll-call lib="C:/LVDemo x86/toupcam.dll" fn="Toupcam_put_ExpoTime"("htoucpam"=w219, "Time"=5000) -> ()  [unwired: 6 in, 2 out]
          n174 = property on="Expotime" class="Slide (strict)"("Scale.Minimum"=w234, "Scale.Maximum"=w233, "Value"=w232) -> ()  [unwired: 2 in, 2 out]
          n175 = property on="Expotime 2" class="Slide (严格)"("Scale.Minimum"=w207, "Scale.Maximum"=w206, "Value"=w205) -> ()  [unwired: 2 in, 2 out]
          n176 = property on="ExpoGain" class="Slide (严格)"("Scale.Minimum"=w241, "Scale.Maximum"=w240, "Value"=w239) -> ()  [unwired: 2 in, 2 out]
          n177 = property on="ExpoGain 2" class="Slide (严格)"("Scale.Minimum"=w204, "Scale.Maximum"=w203, "Value"=w202) -> ()  [unwired: 2 in, 2 out]
          n178 = dll-call lib="C:/LVDemo x86/toupcam.dll" fn="Toupcam_get_ResolutionNumber"("htoucpam"=w197) -> ("返回类型"=w194:u32, "htoucpam"=w193:i32)  [unwired: 3 in, 2 out]
          n179 = dll-call lib="C:/LVDemo x86/toupcam.dll" fn="Toupcam_get_ResolutionNumber"("htoupcam"=w219) -> ("返回类型"=w224:u32, "htoupcam"=w223:i32)  [unwired: 3 in, 2 out]
          n180 = for {
            N: w224 -> [_]
            tunnel: w223 -> [w275]
            tunnel: [w266] -> w222 mode=indexing
            i -> [w267]
            # "Enum Res"
            n181 = dll-call lib="C:/LVDemo x86/toupcam.dll" fn="Toupcam_get_Resolution"("htoupcam"=w275, "ResNum"=w267, "pWidth"="width12", "pHeight"="height12") -> ("pWidth"=w269:i32, "pHeight"=w268:i32)  [unwired: 6 in, 2 out]
            n182 = Number To Decimal String(number=w269) -> (decimal integer string=w270:string)  [unwired: 1 in]
            n183 = Number To Decimal String(number=w268) -> (decimal integer string=w272:string)  [unwired: 1 in]
            n184 = Concatenate Strings(w270, "*", w272) -> (w266:string)
          }
          n185 = for {
            N: w194 -> [_]
            tunnel: w193 -> [w263]
            tunnel: [w256] -> w191 mode=indexing
            i -> [w257]
            # "Enum Res"
            n186 = dll-call lib="C:/LVDemo x86/toupcam.dll" fn="Toupcam_get_Resolution"("htoupcam"=w263, "ResNum"=w257, "pWidth"="width22", "pHeight"="height22") -> ("pWidth"=w259:i32, "pHeight"=w258:i32)  [unwired: 6 in, 2 out]
            n187 = Number To Decimal String(number=w259) -> (decimal integer string=w260:string)  [unwired: 1 in]
            n188 = Number To Decimal String(number=w258) -> (decimal integer string=w262:string)  [unwired: 1 in]
            n189 = Concatenate Strings(w260, "*", w262) -> (w256:string)
          }
          n190 = dll-call lib="C:/LVDemo x86/toupcam.dll" fn="Toupcam_get_Resolution"("htoupcam"=w193, "ResNum"="Live Resolution 2", "pWidth"="Width 2", "pHeight"="Height 2") -> ("htoupcam"=w184:i32, "pWidth"=w215:i32, "pHeight"=w214:i32)  [unwired: 5 in, 2 out]
          n191 = dll-call lib="C:/LVDemo x86/toupcam.dll" fn="Toupcam_put_eSize"("htoupcam"=w193, "nResolutionIndex"="Live Resolution 2") -> ()  [unwired: 6 in, 2 out]
          n192 = dll-call lib="C:/LVDemo x86/toupcam.dll" fn="Toupcam_get_Resolution"("htoupcam"=w223, "ResNum"="Live Resolution", "pWidth"="Width", "pHeight"="Height") -> ("htoupcam"=w216:i32, "pWidth"=w242:i32, "pHeight"=w243:i32)  [unwired: 5 in, 2 out]
          n193 = dll-call lib="C:/LVDemo x86/toupcam.dll" fn="Toupcam_put_eSize"("htoupcam"=w223, "nResolutionIndex"="Live Resolution") -> ()  [unwired: 6 in, 2 out]
          n194 = property on="Live Resolution" class="Ring (严格)"("Strings []"=w222) -> ()  [unwired: 2 in, 2 out]
          n195 = property on="Still Image Resolution" class="Ring (严格)"("Strings []"=w222) -> ()  [unwired: 2 in, 2 out]
          n196 = property on="Live Resolution 2" class="Ring (严格)"("Strings []"=w191) -> ()  [unwired: 2 in, 2 out]
          n197 = property on="Still Image Resolution 2" class="Ring (严格)"("Strings []"=w191) -> ()  [unwired: 2 in, 2 out]
          n198 = Bundle("pWidth"=w242, "pHeight"=w243) -> (w231:cluster{"pWidth":i32, "pHeight":i32})  [unwired: 1 in]
          n199 = Bundle("pWidth"=w215, "pHeight"=w214) -> (w213:cluster{"pWidth":i32, "pHeight":i32})  [unwired: 1 in]
          n200 = dll-call lib="C:/LVDemo x86/toupcam.dll" fn="Toupcam_get_Mode"("htoupcam"=w184, "bMode"="Mode 2") -> ("返回类型"=w186:i32)  [unwired: 5 in, 2 out]
          n201 = dll-call lib="C:/LVDemo x86/toupcam.dll" fn="Toupcam_get_Mode"("htoupcam"=w216, "bMode"="Mode") -> ("返回类型"=w218:i32)  [unwired: 5 in, 2 out]
          n202 = dll-call lib="C:/LVDemo x86/toupcam.dll" fn="Toupcam_get_MonoMode"("htoupcam"=w184) -> ("返回类型"=w187:i32)  [unwired: 4 in, 2 out]
          n203 = dll-call lib="C:/LVDemo x86/toupcam.dll" fn="Toupcam_get_MonoMode"("htoupcam"=w216) -> ("返回类型"=w225:i32)  [unwired: 4 in, 2 out]
          n204 = dll-call lib="C:/LVDemo x86/toupcam.dll" fn="Toupcam_get_MaxSpeed"("htoupcam"=w184) -> ("返回类型"=w189:u8)  [unwired: 4 in, 2 out]
          n205 = dll-call lib="C:/LVDemo x86/toupcam.dll" fn="Toupcam_get_Speed"("htoupcam"=w184, "speed"="speed 2") -> ("speed"=w190:u8)  [unwired: 5 in, 2 out]
          n206 = dll-call lib="C:/LVDemo x86/toupcam.dll" fn="Toupcam_get_MaxSpeed"("htoupcam"=w216) -> ("返回类型"=w227:u8)  [unwired: 4 in, 2 out]
          n207 = dll-call lib="C:/LVDemo x86/toupcam.dll" fn="Toupcam_get_Speed"("htoupcam"=w216, "speed"="speed") -> ("speed"=w228:u8)  [unwired: 5 in, 2 out]
          n208 = Equal To 0?(x=w186) -> (x = 0?=w185:bool)
          n209 = Equal To 0?(x=w218) -> (x = 0?=w217:bool)
          n210 = case shown="1" w187 {
            frame 0, Default {
              w252 = T3."Disabled and Grayed Out" ("禁用")
              # "Mono"
              n211 = property on="Brightness 2" class="Slide (严格)"("DisabledEnum"=w252) -> ()  [unwired: 2 in, 2 out]
              n212 = property on="Contrast 2" class="Slide (严格)"("DisabledEnum"=w252) -> ()  [unwired: 2 in, 2 out]
              n213 = property on="Gamma 2" class="Slide (严格)"("DisabledEnum"=w252) -> ()  [unwired: 2 in, 2 out]
              n214 = property on="Saturation 2" class="Slide (严格)"("DisabledEnum"=w252) -> ()  [unwired: 2 in, 2 out]
              n215 = property on="Hue 2" class="Slide (严格)"("DisabledEnum"=w252) -> ()  [unwired: 2 in, 2 out]
              n216 = property on="AutoWB 2" class="Bool"("DisabledEnum"=w252) -> ()  [unwired: 2 in, 2 out]
              n217 = property on="Color Default 2" class="Bool"("DisabledEnum"=w252) -> ()  [unwired: 2 in, 2 out]
              n218 = property on="Temp 2" class="Slide (严格)"("DisabledEnum"=w252) -> ()  [unwired: 2 in, 2 out]
              n219 = property on="WBDefault 2" class="Bool"("DisabledEnum"=w252) -> ()  [unwired: 2 in, 2 out]
              n220 = property on="Tint 2" class="Slide (严格)"("DisabledEnum"=w252) -> ()  [unwired: 2 in, 2 out]
            }
            frame 1 {
              w253 = T3."Enabled" ("禁用")
              # "Mono"
              n221 = property on="Brightness 2" class="Slide (严格)"("DisabledEnum"=w253) -> ()  [unwired: 2 in, 2 out]
              n222 = property on="Contrast 2" class="Slide (严格)"("DisabledEnum"=w253) -> ()  [unwired: 2 in, 2 out]
              n223 = property on="Gamma 2" class="Slide (严格)"("DisabledEnum"=w253) -> ()  [unwired: 2 in, 2 out]
              n224 = property on="Saturation 2" class="Slide (严格)"("DisabledEnum"=w253) -> ()  [unwired: 2 in, 2 out]
              n225 = property on="Hue 2" class="Slide (严格)"("DisabledEnum"=w253) -> ()  [unwired: 2 in, 2 out]
              n226 = property on="AutoWB 2" class="Bool"("DisabledEnum"=w253) -> ()  [unwired: 2 in, 2 out]
              n227 = property on="Color Default 2" class="Bool"("DisabledEnum"=w253) -> ()  [unwired: 2 in, 2 out]
              n228 = property on="Temp 2" class="Slide (严格)"("DisabledEnum"=w253) -> ()  [unwired: 2 in, 2 out]
              n229 = property on="WBDefault 2" class="Bool"("DisabledEnum"=w253) -> ()  [unwired: 2 in, 2 out]
              n230 = property on="Tint 2" class="Slide (严格)"("DisabledEnum"=w253) -> ()  [unwired: 2 in, 2 out]
            }
          }
          n231 = case shown="1" w225 {
            frame 0, Default {
              w276 = T3."Disabled and Grayed Out" ("禁用")
              # "Mono"
              n232 = property on="Brightness" class="Slide (严格)"("DisabledEnum"=w276) -> ()  [unwired: 2 in, 2 out]
              n233 = property on="Hue" class="Slide (严格)"("DisabledEnum"=w276) -> ()  [unwired: 2 in, 2 out]
              n234 = property on="Contrast" class="Slide (严格)"("DisabledEnum"=w276) -> ()  [unwired: 2 in, 2 out]
              n235 = property on="Gamma" class="Slide (严格)"("DisabledEnum"=w276) -> ()  [unwired: 2 in, 2 out]
              n236 = property on="AutoWB" class="Bool"("DisabledEnum"=w276) -> ()  [unwired: 2 in, 2 out]
              n237 = property on="Temp" class="Slide (严格)"("DisabledEnum"=w276) -> ()  [unwired: 2 in, 2 out]
              n238 = property on="Tint" class="Slide (严格)"("DisabledEnum"=w276) -> ()  [unwired: 2 in, 2 out]
              n239 = property on="Saturation" class="Slide (严格)"("DisabledEnum"=w276) -> ()  [unwired: 2 in, 2 out]
              n240 = property on="WBDefault" class="Bool"("DisabledEnum"=w276) -> ()  [unwired: 2 in, 2 out]
              n241 = property on="Color Default" class="Bool"("DisabledEnum"=w276) -> ()  [unwired: 2 in, 2 out]
            }
            frame 1 {
              w277 = T3."Enabled" ("禁用")
              # "Mono"
              n242 = property on="Brightness" class="Slide (严格)"("DisabledEnum"=w277) -> ()  [unwired: 2 in, 2 out]
              n243 = property on="Hue" class="Slide (严格)"("DisabledEnum"=w277) -> ()  [unwired: 2 in, 2 out]
              n244 = property on="Contrast" class="Slide (严格)"("DisabledEnum"=w277) -> ()  [unwired: 2 in, 2 out]
              n245 = property on="Gamma" class="Slide (严格)"("DisabledEnum"=w277) -> ()  [unwired: 2 in, 2 out]
              n246 = property on="AutoWB" class="Bool"("DisabledEnum"=w277) -> ()  [unwired: 2 in, 2 out]
              n247 = property on="Temp" class="Slide (严格)"("DisabledEnum"=w277) -> ()  [unwired: 2 in, 2 out]
              n248 = property on="Tint" class="Slide (严格)"("DisabledEnum"=w277) -> ()  [unwired: 2 in, 2 out]
              n249 = property on="Saturation" class="Slide (严格)"("DisabledEnum"=w277) -> ()  [unwired: 2 in, 2 out]
              n250 = property on="WBDefault" class="Bool"("DisabledEnum"=w277) -> ()  [unwired: 2 in, 2 out]
              n251 = property on="Color Default" class="Bool"("DisabledEnum"=w277) -> ()  [unwired: 2 in, 2 out]
            }
          }
          n252 = case shown="假" w185 {
            frame True {
              n253 = property on="Bin/Skip Mode 2" class="Bool (严格)"("DisabledEnum"=T3."Enabled" ("禁用")) -> ()  [unwired: 2 in, 2 out]
            }
            frame False {
              n254 = property on="Bin/Skip Mode 2" class="Bool (严格)"("DisabledEnum"=T3."Disabled and Grayed Out" ("禁用")) -> ()  [unwired: 2 in, 2 out]
            }
          }
          n255 = case shown="假" w217 {
            frame True {
              n256 = property on="Bin/Skip Mode" class="Bool (严格)"("DisabledEnum"=T3."Enabled" ("禁用")) -> ()  [unwired: 2 in, 2 out]
            }
            frame False {
              n257 = property on="Bin/Skip Mode" class="Bool (严格)"("DisabledEnum"=T3."Disabled and Grayed Out" ("禁用")) -> ()  [unwired: 2 in, 2 out]
            }
          }
          n258 = property on="Frame Speed 2" class="Slide (严格)"("Value"=w190, "Scale.Maximum"=w189, "Scale.Minimum"=0) -> ()  [unwired: 2 in, 2 out]
          n259 = property on="Frame Speed" class="Slide (严格)"("Value"=w228, "Scale.Maximum"=w227, "Scale.Minimum"=0) -> ()  [unwired: 2 in, 2 out]
        }
        frame #1 {
          w280 = T3."Disabled and Grayed Out" ("禁用")
          w279 = TRUE
          w278 = TRUE
          w285 = TRUE
          w284 = 1000
          w283 = 6503
          w282 = 128
          w281 = 100
          w286 = 0
          # "SetSliderDefault"
          n260 = property on="Gamma" class="Slide (严格)"("Value"=w281) -> ()  [unwired: 2 in, 2 out]
          n261 = property on="Saturation" class="Slide (严格)"("Value"=w282) -> ()  [unwired: 2 in, 2 out]
          n262 = property on="Temp" class="Slide (严格)"("Value"=w283) -> ()  [unwired: 2 in, 2 out]
          n263 = property on="Tint" class="Slide (严格)"("Value"=w284) -> ()  [unwired: 2 in, 2 out]
          n264 = property on="AutoExpo" class="Bool (严格)"("Value"=w285) -> ()  [unwired: 2 in, 2 out]
          n265 = property on="Brightness" class="Slide (严格)"("Value"=w286) -> ()  [unwired: 2 in, 2 out]
          n266 = property on="Contrast" class="Slide (严格)"("Value"=w286) -> ()  [unwired: 2 in, 2 out]
          n267 = property on="Hue" class="Slide (严格)"("Value"=w286) -> ()  [unwired: 2 in, 2 out]
          n268 = property on="Gamma 2" class="Slide (严格)"("Value"=w281) -> ()  [unwired: 2 in, 2 out]
          n269 = property on="Saturation 2" class="Slide (严格)"("Value"=w282) -> ()  [unwired: 2 in, 2 out]
          n270 = property on="Temp 2" class="Slide (严格)"("Value"=w283) -> ()  [unwired: 2 in, 2 out]
          n271 = property on="Tint 2" class="Slide (严格)"("Value"=w284) -> ()  [unwired: 2 in, 2 out]
          n272 = property on="AutoExpo 2" class="Bool (严格)"("Value"=w285) -> ()  [unwired: 2 in, 2 out]
          n273 = property on="Brightness 2" class="Slide (严格)"("Value"=w286) -> ()  [unwired: 2 in, 2 out]
          n274 = property on="Contrast 2" class="Slide (严格)"("Value"=w286) -> ()  [unwired: 2 in, 2 out]
          n275 = property on="Hue 2" class="Slide (严格)"("Value"=w286) -> ()  [unwired: 2 in, 2 out]
          n276 = property on="Bin/Skip Mode" class="Bool (严格)"("Value"=w278) -> ()  [unwired: 2 in, 2 out]
          n277 = property on="Chrome/Mono" class="Bool (严格)"("Value"=w279) -> ()  [unwired: 2 in, 2 out]
          n278 = property on="Expotime" class="Slide (strict)"("DisabledEnum"=w280) -> ()  [unwired: 2 in, 2 out]
          n279 = property on="ExpoGain" class="Slide (strict)"("DisabledEnum"=w280) -> ()  [unwired: 2 in, 2 out]
          n280 = property on="Expotime 2" class="Slide (严格)"("DisabledEnum"=w280) -> ()  [unwired: 2 in, 2 out]
          n281 = property on="ExpoGain 2" class="Slide (严格)"("DisabledEnum"=w280) -> ()  [unwired: 2 in, 2 out]
          n282 = property on="Bin/Skip Mode 2" class="Bool (严格)"("Value"=w278) -> ()  [unwired: 2 in, 2 out]
          n283 = property on="Chrome/Mono 2" class="Bool (严格)"("Value"=w279) -> ()  [unwired: 2 in, 2 out]
          n284 = property class="TabCtl (严格)"("Visible"=FALSE) -> ()  [unwired: 2 in, 2 out]
        }
        frame #2 {
          w292 = u32 0  # Event2
          w295 = u32 0  # Event1
          w297 = T4 4 items=["Grayscale (U8)", "Grayscale (I16)", "Grayscale (SGL)", "Complex (CSG)", "RGB (U32)", "HSL (U32)", "RGB (U64)", "Grayscale (U16)"] ("Image Type")
          w306 = T4 4 items=["Grayscale (U8)", "Grayscale (I16)", "Grayscale (SGL)", "Complex (CSG)", "RGB (U32)", "HSL (U32)", "RGB (U64)", "Grayscale (U16)"] ("Image Type")
          n285 = Create User Event(user event datatype=w295) -> (user event=w294:refnum<user-event>)  [unwired: 1 in, 1 out]
          n286 = Create User Event(user event datatype=w292) -> (user event=w291:refnum<user-event>)  [unwired: 1 in, 1 out]
          n287 = call "IMAQ Create"("Image Name"="", "Image Type"=w306) -> ("New Image"=w307:T2)  [unwired: 3 in, 1 out]
          n288 = call "IMAQ Create"("Image Name"="", "Image Type"=w297) -> ("New Image"=w296:T2)  [unwired: 3 in, 1 out]
          n289 = register-events(w294) -> (reference out=w293:refnum<event-registration>)  [unwired: 2 in, 1 out]
          n290 = register-events(w291) -> (reference out=w290:refnum<event-registration>)  [unwired: 2 in, 1 out]
          n291 = dll-call lib="C:/LVDemo x86/toupcam_labview.dll" fn="Start"(error in=w304, "htoupcam"=w309, "rewr"=w294) -> (error out=w303:errorcluster, "htoupcam"=w302:i32)  [unwired: 4 in, 1 out]
          n292 = dll-call lib="C:/LVDemo x86/toupcam_labview.dll" fn="Start"("htoupcam"=w301, "rewr"=w291) -> ("htoupcam"=w300:i32)  [unwired: 5 in, 2 out]
          n293 = while {
            tunnel: w302 -> [w315]
            tunnel: w307 -> [w319]
            tunnel: w305 -> [w318]
            tunnel: w300 -> [w311]
            tunnel: w299 -> [w317]
            tunnel: w296 -> [w310]
            tunnel: w293 -> [w316]
            tunnel: w290 -> [w314]
            tunnel: [w313] -> w289
            tunnel: [w312] -> w288
            stop <- "Stop" stop-if-true
            n294 = event shown="[2] 应用程序实例关闭" {
              selector: w316 -> [_ _ _]
              dyn-events: _ -> [_ _ _]
              timeout: _ -> [_ _ _]
              tunnel: w319 -> [_ w372 w420]
              tunnel: w318 -> [_ w371 _]
              tunnel: w315 -> [_ w369 w418]
              tunnel: [_ w368 _] -> w312
              tunnel: w311 -> [_ _ w416]
              tunnel: w310 -> [_ _ w419]
              event Timeout {
                n295 = event-data() -> ()  [unwired: 1 in, 2 out]
              }
              event User Event {
                n296 = event-data() -> ("Event1"=w370:u32)  [unwired: 1 in]
                n297 = case shown="5" w370 {
                  tunnel: w372 -> [w376 w391 _ _ _]
                  tunnel: w371 -> [w380 _ _ _ _]
                  tunnel: w369 -> [w375 w386 w405 w410 _]
                  tunnel: [w373 w385 _ _ _] -> w368
                  frame 4, Default {
                    # "ShowVideo"
                    n298 = Unbundle(w380) -> ("pWidth"=w378:i32, "pHeight"=w377:i32)
                    n299 = Multiply(x=w378, y=w377) -> (x*y=w382:i32)
                    n300 = Initialize Array(u32 0, w382) -> (w379:u32[])
                    n301 = dll-call lib="C:/LVDemo x86/toupcam.dll" fn="Toupcam_PullImage"("htoupcam"=w375, "pImageData"=w379, "bits"=32, "nWidth"=w378, "nHeight"=w377) -> ("pImageData"=w384:u32[])  [unwired: 8 in, 2 out]
                    n302 = Reshape Array(w384, w377, w378) -> (w383:u32[][])
                    n303 = call "IMAQ ArrayToColorImage"("Image Pixels (U32)"=w383, "Image"=w376) -> ("Image Out"=w373:T2)  [unwired: 3 in, 1 out]
                    n304 = local write "Video"(w373) -> ()
                  }
                  frame 5 {
                    # "Capture still Image"
                    n305 = property on="Still Image Resolution" class="Ring (严格)"() -> ("Value"=w387:u16)  [unwired: 2 in, 2 out]
                    n306 = dll-call lib="C:/LVDemo x86/toupcam.dll" fn="Toupcam_get_StillResolution"("htoupcam"=w386, "nIndex"=w387, "pWidth"="Still_Width 3", "pHeight"="Still_Height 3") -> ("htoupcam"=w403:i32, "pWidth"=w389:i32, "pHeight"=w390:i32)  [unwired: 5 in, 2 out]
                    n307 = Multiply(x=w389, y=w390) -> (x*y=w388:i32)
                    n308 = Initialize Array(u32 0, w388) -> (w402:u32[])
                    n309 = dll-call lib="C:/LVDemo x86/toupcam.dll" fn="Toupcam_PullStillImage"("htoupcam"=w403, "pImageData"=w402, "bits"=32, "pnWidth"=w389, "pnHeight"=w390) -> ("pImageData"=w400:u32[])  [unwired: 8 in, 2 out]
                    n310 = Reshape Array(w400, w390, w389) -> (w392:u32[][])
                    n311 = call "IMAQ ArrayToColorImage"("Image Pixels (U32)"=w392, "Image"=w391) -> ("Image Out"=w385:T2)  [unwired: 3 in, 1 out]
                    n312 = Format Date/Time String(time format string (%c)="%Y-%m-%d %H：%M：%S.bmp ") -> (date/time string=w396:string)  [unwired: 2 in]
                    n313 = Concatenate Strings("D:\\Captured Image\\", w396) -> (w393:string)
                    n314 = String To Path(string=w393) -> (path=w395:path)
                    n315 = call-poly "IMAQ Write File 2"("File Path"=w395, "Image"=w385) -> ()  [unwired: 8 in, 2 out]
                  }
                  frame 1 {
                    # "Auto Expo"
                    n316 = dll-call lib="C:/LVDemo x86/toupcam.dll" fn="Toupcam_get_ExpoAGain"("htoupcam"=w405, "ExpoGain"="ExpoGain 5") -> ("ExpoGain"=w406:u16)  [unwired: 5 in, 2 out]
                    n317 = dll-call lib="C:/LVDemo x86/toupcam.dll" fn="Toupcam_get_ExpoTime"("htoupcam"=w405, "Expotime"="Expotime 5") -> ("Expotime"=w407:u32)  [unwired: 5 in, 2 out]
                    n318 = property on="ExpoGain" class="Slide (严格)"("Value"=w406) -> ()  [unwired: 2 in, 2 out]
                    n319 = property on="Expotime" class="Slide (严格)"("Value"=w407) -> ()  [unwired: 2 in, 2 out]
                  }
                  frame 2 {
                    # "Auto WhiteBalance"
                    n320 = dll-call lib="C:/LVDemo x86/toupcam.dll" fn="Toupcam_get_TempTint"("htoupcam"=w410, "Temp"="Temp 5", "Tint"="Tint 5") -> ("Temp"=w412:i32, "Tint"=w411:i32)  [unwired: 5 in, 2 out]
                    n321 = property on="Tint" class="Slide (严格)"("Value"=w411) -> ()  [unwired: 2 in, 2 out]
                    n322 = property on="Temp" class="Slide (严格)"("Value"=w412) -> ()  [unwired: 2 in, 2 out]
                  }
                  frame 3 {
                  }
                }
              }
              event Application Instance Close {
                n323 = event-data() -> ()  [unwired: 1 in, 1 out]
                n324 = call "IMAQ Dispose"("Image"=w420) -> ()  [unwired: 5 in, 1 out]
                n325 = call "IMAQ Dispose"("Image"=w419) -> ()  [unwired: 5 in, 1 out]
                n326 = dll-call lib="C:/LVDemo x86/toupcam.dll" fn="Toupcam_Stop"("htoupcam2"=w416) -> ("htoupcam2"=w415:i32)  [unwired: 4 in, 2 out]
                n327 = dll-call lib="C:/LVDemo x86/toupcam.dll" fn="Toupcam_Stop"("htoucpam1"=w418) -> ("htoucpam1"=w417:i32)  [unwired: 4 in, 2 out]
                n328 = dll-call lib="C:/LVDemo x86/toupcam.dll" fn="Toupcam_Close"("htoupcam2"=w415) -> ()  [unwired: 5 in, 2 out]
                n329 = dll-call lib="C:/LVDemo x86/toupcam.dll" fn="Toupcam_Close"("htoupcam1"=w417) -> ()  [unwired: 5 in, 2 out]
              }
            }
            n330 = event shown="[1] <Event2>: 用户事件" {
              selector: w314 -> [_ _]
              dyn-events: _ -> [_ _]
              timeout: _ -> [_ _]
              tunnel: w317 -> [_ w325]
              tunnel: w310 -> [_ w324]
              tunnel: w311 -> [_ w322]
              tunnel: [_ w321] -> w313
              event Timeout {
                n331 = event-data() -> ()  [unwired: 1 in, 2 out]
              }
              event User Event {
                n332 = event-data() -> ("Event2"=w323:u32)  [unwired: 1 in]
                n333 = case shown="5" w323 {
                  tunnel: w325 -> [_ _ w347 _]
                  tunnel: w324 -> [_ _ w338 w353]
                  tunnel: w322 -> [w326 w331 w337 w349]
                  tunnel: [_ _ w336 w348] -> w321
                  frame 1 {
                    n334 = dll-call lib="C:/LVDemo x86/toupcam.dll" fn="Toupcam_get_ExpoAGain"("htoupcam"=w326, "ExpoGain"="ExpoGain 6") -> ("ExpoGain"=w328:u16)  [unwired: 5 in, 2 out]
                    n335 = dll-call lib="C:/LVDemo x86/toupcam.dll" fn="Toupcam_get_ExpoTime"("htoupcam"=w326, "Expotime"="Expotime 6") -> ("Expotime"=w327:u32)  [unwired: 5 in, 2 out]
                    n336 = property on="Expotime 2" class="Slide (严格)"("Value"=w327) -> ()  [unwired: 2 in, 2 out]
                    n337 = property on="ExpoGain 2" class="Slide (严格)"("Value"=w328) -> ()  [unwired: 2 in, 2 out]
                  }
                  frame 2 {
                    n338 = dll-call lib="C:/LVDemo x86/toupcam.dll" fn="Toupcam_get_TempTint"("htoupcam"=w331, "Temp"="Temp 6", "Tint"="Tint 6") -> ("Temp"=w332:i32, "Tint"=w333:i32)  [unwired: 5 in, 2 out]
                    n339 = property on="Temp 2" class="Slide (严格)"("Value"=w332) -> ()  [unwired: 2 in, 2 out]
                    n340 = property on="Tint 2" class="Slide (严格)"("Value"=w333) -> ()  [unwired: 2 in, 2 out]
                  }
                  frame 4, Default {
                    n341 = Unbundle(w347) -> ("pWidth"=w341:i32, "pHeight"=w342:i32)
                    n342 = Multiply(x=w341, y=w342) -> (x*y=w346:i32)
                    n343 = Initialize Array(u32 0, w346) -> (w344:u32[])
                    n344 = dll-call lib="C:/LVDemo x86/toupcam.dll" fn="Toupcam_PullImage"("htoupcam"=w337, "pImageData"=w344, "bits"=32, "nWidth"=w341, "nHeight"=w342) -> ("pImageData"=w340:u32[])  [unwired: 8 in, 2 out]
                    n345 = Reshape Array(w340, w342, w341) -> (w339:u32[][])
                    n346 = call "IMAQ ArrayToColorImage"("Image Pixels (U32)"=w339, "Image"=w338) -> ("Image Out"=w336:T2)  [unwired: 3 in, 1 out]
                    n347 = local write "Video 2"(w336) -> ()
                  }
                  frame 5 {
                    # "Capture still Image"
                    n348 = property on="Still Image Resolution 2" class="Ring (严格)"() -> ("Value"=w350:u16)  [unwired: 2 in, 2 out]
                    n349 = dll-call lib="C:/LVDemo x86/toupcam.dll" fn="Toupcam_get_StillResolution"("htoupcam"=w349, "nIndex"=w350, "pWidth"="Still_Width 4", "pHeight"="Still_Height 4") -> ("htoupcam"=w366:i32, "pWidth"=w355:i32, "pHeight"=w356:i32)  [unwired: 5 in, 2 out]
                    n350 = Multiply(x=w355, y=w356) -> (x*y=w354:i32)
                    n351 = Initialize Array(u32 0, w354) -> (w365:u32[])
                    n352 = dll-call lib="C:/LVDemo x86/toupcam.dll" fn="Toupcam_PullStillImage"("htoupcam"=w366, "pImageData"=w365, "bits"=32, "pnWidth"=w355, "pnHeight"=w356) -> ("pImageData"=w363:u32[])  [unwired: 8 in, 2 out]
                    n353 = Reshape Array(w363, w356, w355) -> (w357:u32[][])
                    n354 = call "IMAQ ArrayToColorImage"("Image Pixels (U32)"=w357, "Image"=w353) -> ("Image Out"=w348:T2)  [unwired: 3 in, 1 out]
                    n355 = Format Date/Time String(time format string (%c)="%Y-%m-%d %H：%M：%S.bmp ") -> (date/time string=w361:string)  [unwired: 2 in]
                    n356 = Concatenate Strings("D:\\Captured Image\\", w361) -> (w358:string)
                    n357 = String To Path(string=w358) -> (path=w360:path)
                    n358 = call-poly "IMAQ Write File 2"("File Path"=w360, "Image"=w348) -> ()  [unwired: 8 in, 2 out]
                  }
                }
              }
            }
          }
          n359 = call "IMAQ Dispose"("Image"=w288) -> ()  [unwired: 5 in, 1 out]
          n360 = call "IMAQ Dispose"("Image"=w289) -> ()  [unwired: 5 in, 1 out]
        }
        frame #3 {
          n361 = dll-call lib="C:/LVDemo x86/toupcam.dll" fn="Toupcam_Stop"("参数1"=w421) -> ()  [unwired: 5 in, 2 out]
          n362 = dll-call lib="C:/LVDemo x86/toupcam.dll" fn="Toupcam_Stop"("参数1"=w422) -> ()  [unwired: 5 in, 2 out]
        }
        frame #4 {
          n363 = dll-call lib="C:/LVDemo x86/toupcam.dll" fn="Toupcam_Close"(error in=w425, "参数1"=w426) -> ()  [unwired: 4 in, 2 out]
          n364 = dll-call lib="C:/LVDemo x86/toupcam.dll" fn="Toupcam_Close"("参数1"=w423) -> ()  [unwired: 5 in, 2 out]
          n365 = Stop(stop? (T)=TRUE) -> ()
        }
      }
    }
    frame Error {
    }
  }
